vi "WPI_MotorControlSafetyCheck.vi"(0 "MotorControlDevRef":T1={"DeviceStatus"={"status"=FALSE, "code"=0, "source"=""}, "Type"=enum."PWM", "PWM"={"PWM Channel"=enum."Invalid", "DeadBand"={"Name"="", "maxPositivePwm"=0, "minPositivePwm"=0, "centerPwm"=0, "maxNegativePwm"=0, "minNegativePwm"=0, "angularRange"=0}}, "CAN"={"Device Number"=0, "SetOutput VI Ref"=variant(refnum<vi> refnum), "GetOutput VI Ref"=variant(refnum<vi> refnum), "Enable VI Ref"=variant(refnum<vi> refnum), "Disable VI Ref"=variant(refnum<vi> refnum), "Data"=variant}, "Invert"=FALSE, "DIO PWM"={"PWM \"Enable\" Channel"=enum."Invalid", "DIOChannel"=enum."Invalid", "PWM Rate"=0.0}}, 5 "menu":T6, 7 "VI Refnum":refnum<vi>, 9 "timeout (ms)":u32=100, 11 "error in (no error)":errorcluster) -> (15 "error out":errorcluster)   [LabVIEW 2025]
doc: "This subVI holds an array of DevRefs, timeout values, and latest update times. These values can be added, updated, tested, and removed.\n\nThis gets called by Open to add a set of values. It gets called by Drive to update the 'last update value'. It gets called by Close to remove a set of values.\n\nIt also gets called by Safety Test via the SafetyCheckEngine that runs as a background task called by the Start Communication loop to test all sets of values for a timeout condition.\n\nThis software is licensed. Open the labview\\readme\\WPI Robotics Library Open Source License.txt file for more information."
uses:
  <vilib>/Rock Robotics/WPI/SafetyOutput/WPI_SafetyOutputCheckMenu.ctl
  <vilib>/Rock Robotics/WPI/MotorControl/WPI_MotorControlDeviceRef.ctl
  <vilib>/Rock Robotics/WPI/MotorControl/WPI_MotorControlType.ctl
  <vilib>/Rock Robotics/SystemInterfaces/DIO/FPGA_DIOPWMChannel.ctl
  <vilib>/Rock Robotics/WPI/PWM/WPI_PWMDeadband.ctl
  <vilib>/Rock Robotics/SystemInterfaces/DIO/FPGA_DIOChannel.ctl
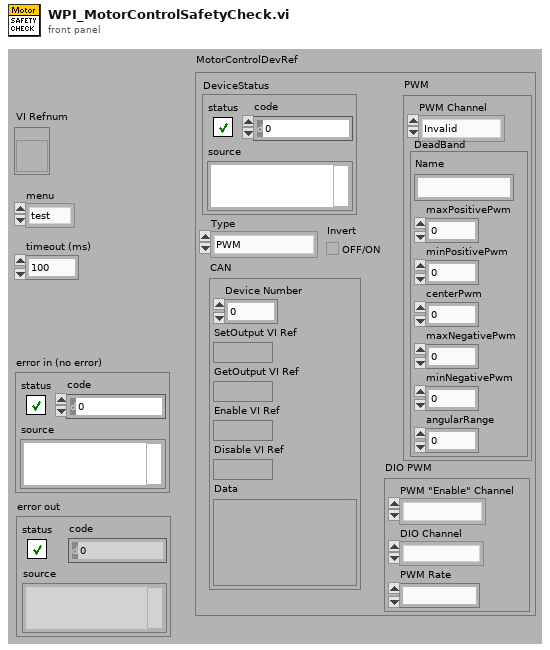
[diagram p1: front panel]
types:
  T1 = typedef "WPI_MotorControlDeviceRef.ctl" = cluster{"DeviceStatus":errorcluster, "Type":T2, "PWM":cluster{"PWM Channel":T3, "DeadBand":T4}, "CAN":cluster{"Device Number":u8, "SetOutput VI Ref":variant, "GetOutput VI Ref":variant, "Enable VI Ref":variant, "Disable VI Ref":variant, "Data":variant}, "Invert":bool, "DIO PWM":cluster{"PWM \"Enable\" Channel":T3, "DIOChannel":T5, "PWM Rate":dbl}}
  T2 = typedef "WPI_MotorControlType.ctl" = enum16{"PWM", "CAN", "DIO PWM"}
  T3 = typedef "FPGA_DIOPWMChannel.ctl" = enum8{"PWM 0", "PWM 1", "PWM 2", "PWM 3", "PWM 4", "PWM 5", "PWM 6", "PWM 7", "PWM 8", "PWM 9", "PWM MXP 0", "PWM MXP 1", "PWM MXP 2", "PWM MXP 3", "PWM MXP 4", "PWM MXP 5", "PWM MXP 6", "PWM MXP 7", "PWM MXP 8", "PWM MXP 9", "Invalid"}
  T4 = typedef "WPI_PWMDeadband.ctl" = cluster{"Name":string, "maxPositivePwm":i32, "minPositivePwm":i32, "centerPwm":i32, "maxNegativePwm":i32, "minNegativePwm":i32, "angularRange":u16}
  T5 = typedef "FPGA_DIOChannel.ctl" = enum8{"DIO 0", "DIO 1", "DIO 2", "DIO 3", "DIO 4", "DIO 5", "DIO 6", "DIO 7", "DIO 8", "DIO 9", "DIO MXP 0", "DIO MXP 1", "DIO MXP 2", "DIO MXP 3", "DIO MXP 4", "DIO MXP 5", "DIO MXP 6", "DIO MXP 7", "DIO MXP 8", "DIO MXP 9", "DIO MXP 10", "DIO MXP 11", "DIO MXP 12", "DIO MXP 13", "DIO MXP 14", "DIO MXP 15", "SPI Port CS1", "SPI Port CS2", "SPI Port CS3", "SPI Port MISO", "SPI Port MOSI", "Invalid"}
  T6 = typedef "WPI_SafetyOutputCheckMenu.ctl" = enum16{"test", "add", "remove", "update"}
  T7 = typedef "WPI_PWMDeviceRef.ctl" = cluster{"DeviceStatus":errorcluster, "PWM Channel":T3}
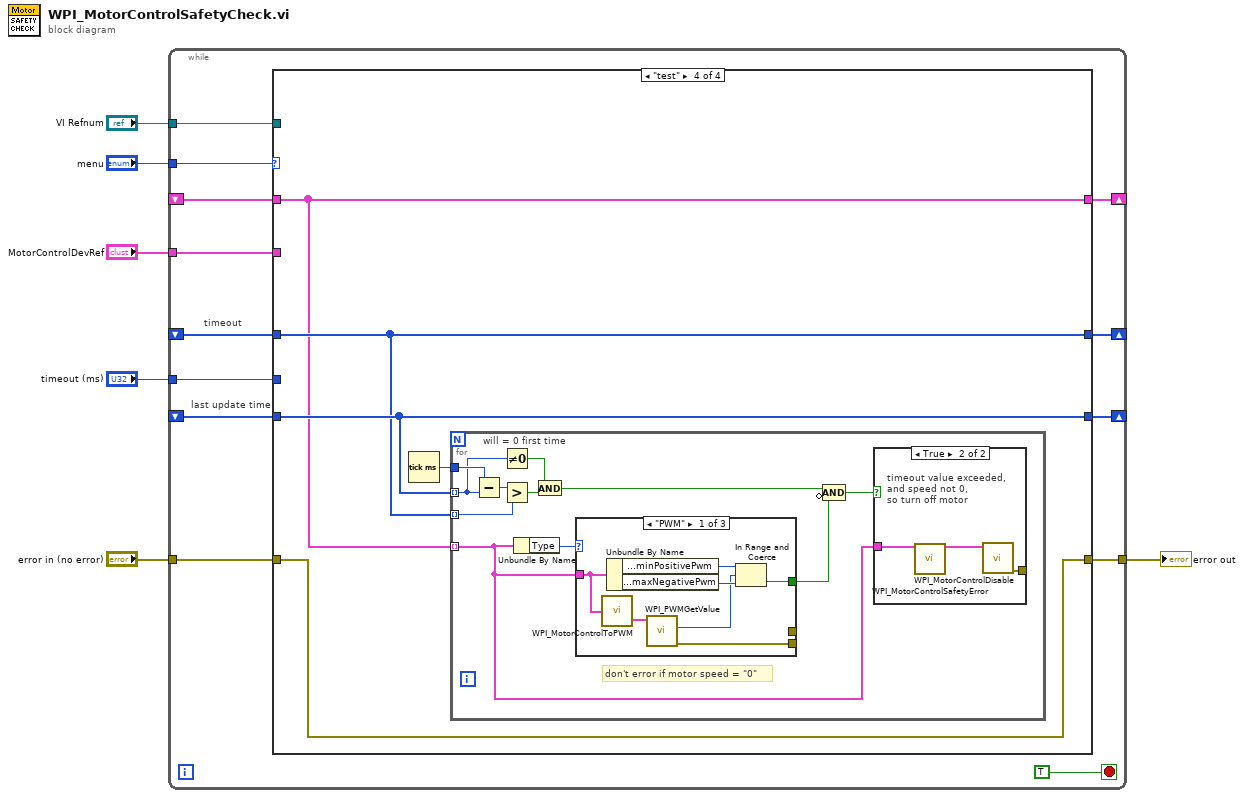
[diagram p0: block diagram]
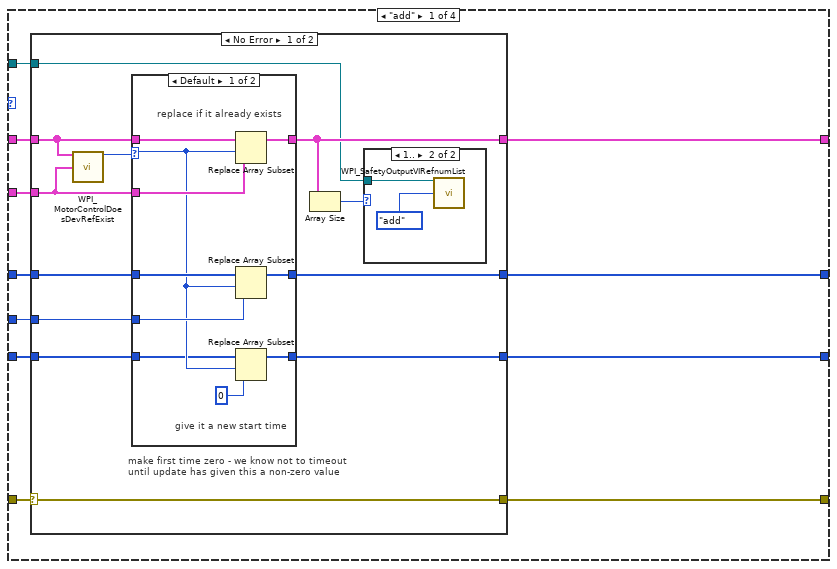
[diagram p2: hidden frame]
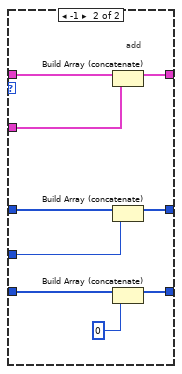
[diagram p4: hidden frame]
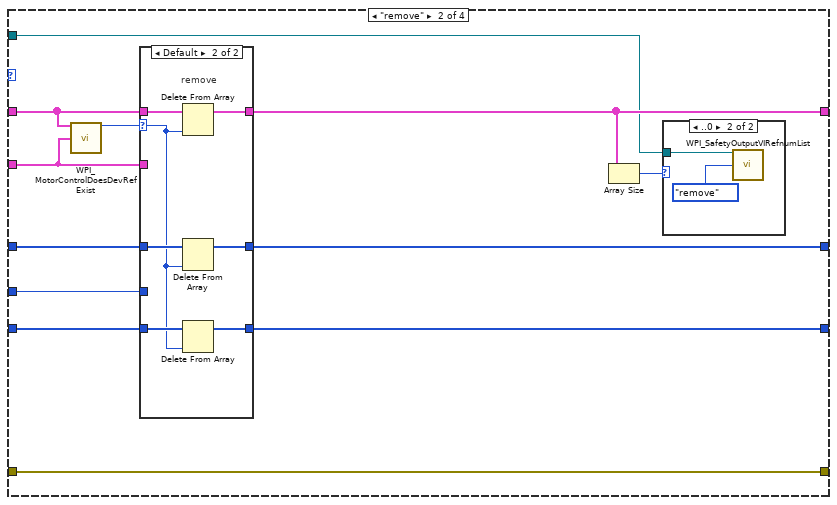
[diagram p6: hidden frame]
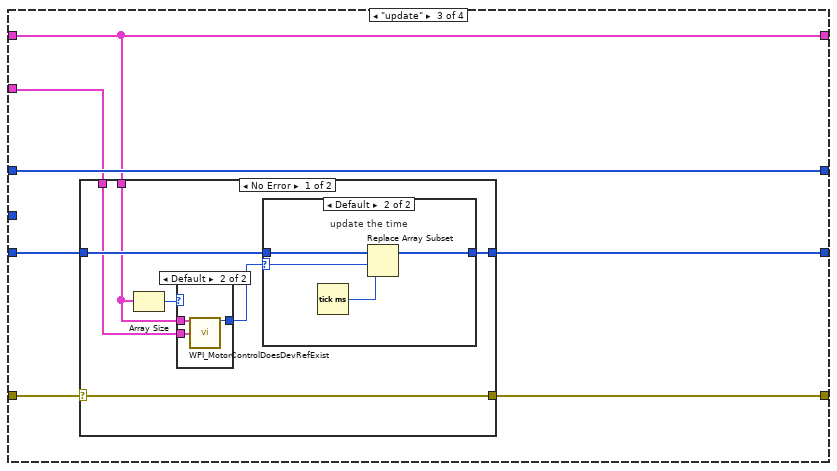
[diagram p9: hidden frame]
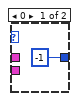
[diagram p10: hidden frame]
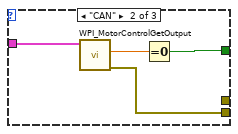
[diagram p13: hidden frame]
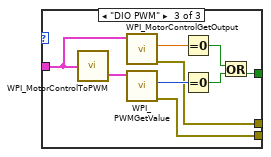
[diagram p14: hidden frame]
diagram:
  n1 = while {
    tunnel: "menu" -> [w18]
    shift-right: [w17] -> _
    shift-left: _ -> [w13]
    tunnel: "MotorControlDevRef" -> [w12]
    shift-right: [w14] -> _
    shift-left: _ -> [w16]
    tunnel: "timeout (ms)" -> [w15]
    shift-right: [w10] -> _
    shift-left: _ -> [w11]
    tunnel: "VI Refnum" -> [w9]
    tunnel: "error in (no error)" -> [w8]
    tunnel: [w7] -> w1
    stop <- TRUE stop-if-true
    # "last update time"
    # "timeout"
    n2 = case shown="\"test\"" w18 {
      tunnel: w13 -> [w30 w69 w93 w117]
      tunnel: [w23 w73 w93 w117] -> w17
      tunnel: w12 -> [w29 w68 w92 _]
      tunnel: w16 -> [w28 w79 w98 w119]
      tunnel: w15 -> [w27 w78 _ _]
      tunnel: [w26 w77 w98 w119] -> w14
      tunnel: w11 -> [w25 w76 w97 w120]
      tunnel: [w24 w75 w96 w120] -> w10
      tunnel: w9 -> [w22 w72 _ _]
      tunnel: w8 -> [w21 w71 w95 w118]
      tunnel: [w20 w71 w94 w118] -> w7
      frame "add" {
        n3 = case shown="No Error" w21 {
          selector: w21 -> [w34 w67]
          tunnel: w30 -> [w33 w66]
          tunnel: w29 -> [w31 _]
          tunnel: w28 -> [w42 w65]
          tunnel: w27 -> [w41 _]
          tunnel: [w40 w65] -> w26
          tunnel: w25 -> [w39 w64]
          tunnel: [w38 w64] -> w24
          tunnel: [w37 w66] -> w23
          tunnel: w22 -> [w36 _]
          tunnel: [w34 w67] -> w20
          frame No Error {
            # "make first time zero - we know not to timeout until update has given this a non-zero value"
            n4 = call <vilib>:"WPI_MotorControlDoesDevRefExist.vi"("MotorControlDeviceRefArray"=w33, "MotorControlDeviceRef"=w31) -> ("index"=w32:i32)  [unwired: 13 out]
            n5 = case shown="Default" w32 {
              selector: w32 -> [w47 _]
              tunnel: w33 -> [w54 w63]
              tunnel: [w53 w62] -> w37
              tunnel: w31 -> [w52 w61]
              tunnel: w42 -> [w51 w60]
              tunnel: w41 -> [w49 w59]
              tunnel: [w50 w58] -> w40
              tunnel: w39 -> [w46 w57]
              tunnel: [w45 w56] -> w38
              frame Default {
                # "give it a new start time"
                # "replace if it already exists"
                n6 = Replace Array Subset(array=w54, new element=w52, index=w47) -> (w53:T1[])
                n7 = Replace Array Subset(array=w51, new element=w49, index=w47) -> (w50:u32[])
                n8 = Replace Array Subset(array=w46, new element=u32 0 ("millisecond timer value"), index=w47) -> (w45:u32[])
              }
              frame -1 {
                # "add"
                n9 = Build Array (concatenate)(w63, w61) -> (w62:T1[])
                n10 = Build Array (concatenate)(w60, w59) -> (w58:u32[])
                n11 = Build Array (concatenate)(w57, u32 0 ("millisecond timer value")) -> (w56:u32[])
              }
            }
            n12 = Array Size(array=w37) -> (size(s)=w35:i32)
            n13 = case shown="1.." w35 {
              tunnel: w36 -> [_ w43]
              frame Default {
              }
              frame 1.. {
                n14 = call <vilib>:"WPI_SafetyOutputVIRefnumList.vi"("VI Refnum"=w43, "menu"=enum16{"read", "add", "remove"}."add") -> ()  [unwired: 14 out]
              }
            }
          }
          frame Error {
            # "do not add if there is an error"
          }
        }
      }
      frame "remove" {
        n15 = call <vilib>:"WPI_MotorControlDoesDevRefExist.vi"("MotorControlDeviceRefArray"=w69, "MotorControlDeviceRef"=w68) -> ("index"=w70:i32)  [unwired: 13 out]
        n16 = case shown="Default" w70 {
          selector: w70 -> [_ w85]
          tunnel: w69 -> [w84 w91]
          tunnel: [w84 w88] -> w73
          tunnel: w68 -> [_ _]
          tunnel: w79 -> [w83 w90]
          tunnel: w78 -> [_ _]
          tunnel: [w83 w87] -> w77
          tunnel: w76 -> [w82 w89]
          tunnel: [w82 w86] -> w75
          frame -1 {
            # "do nothing if it does not exist"
          }
          frame Default {
            # "remove"
            n17 = Delete From Array(array=w91, index=w85) -> (array with subset deleted=w88:T1[])  [unwired: 1 in, 1 out]
            n18 = Delete From Array(array=w90, index=w85) -> (array with subset deleted=w87:u32[])  [unwired: 1 in, 1 out]
            n19 = Delete From Array(array=w89, index=w85) -> (array with subset deleted=w86:u32[])  [unwired: 1 in, 1 out]
          }
        }
        n20 = Array Size(array=w73) -> (size(s)=w74:i32)
        n21 = case shown="..0" w74 {
          tunnel: w72 -> [_ w80]
          frame Default {
          }
          frame ..0 {
            n22 = call <vilib>:"WPI_SafetyOutputVIRefnumList.vi"("VI Refnum"=w80, "menu"=enum16{"read", "add", "remove"}."remove") -> ()  [unwired: 14 out]
          }
        }
      }
      frame "update" {
        n23 = case shown="No Error" w95 {
          selector: w95 -> [w103 w116]
          tunnel: w97 -> [w105 w115]
          tunnel: [w104 w115] -> w96
          tunnel: [w103 w116] -> w94
          tunnel: w93 -> [w100 _]
          tunnel: w92 -> [w99 _]
          frame No Error {
            n24 = Array Size(array=w100) -> (size(s)=w102:i32)
            n25 = case shown="Default" w102 {
              tunnel: w99 -> [_ w109]
              tunnel: [-1 w108] -> w101
              tunnel: w100 -> [_ w107]
              frame 0 {
              }
              frame Default {
                n26 = call <vilib>:"WPI_MotorControlDoesDevRefExist.vi"("MotorControlDeviceRefArray"=w107, "MotorControlDeviceRef"=w109) -> ("index"=w108:i32)  [unwired: 13 out]
              }
            }
            n27 = case shown="Default" w101 {
              selector: w101 -> [_ w111]
              tunnel: w105 -> [w110 w114]
              tunnel: [w110 w113] -> w104
              frame -1 {
                # "don't replace if it doesn't exist"
              }
              frame Default {
                # "update the time"
                n28 = Tick Count (ms)() -> (millisecond timer value=w112:u32)
                n29 = Replace Array Subset(array=w114, new element=w112, index=w111) -> (w113:u32[])
              }
            }
          }
          frame Error {
            # "do not update if there is an error"
          }
        }
      }
      frame "test" {
        n30 = Tick Count (ms)() -> (millisecond timer value=w121:u32)
        n31 = for {
          tunnel: w120 -> [w128] mode=indexing
          tunnel: w121 -> [w132]
          tunnel: w119 -> [w130] mode=indexing
          tunnel: w117 -> [w125] mode=indexing
          # "don't error if motor speed = \"0\""
          # "will = 0 first time"
          n32 = Subtract(x=w132, y=w128) -> (x-y=w131:u32)
          n33 = Not Equal To 0?(x=w128) -> (x != 0?=w127:bool)
          n34 = Greater?(x=w131, y=w130) -> (0:w129:bool)
          n35 = Unbundle By Name(w125) -> ("Type"=w126:T2)
          n36 = And(x=w127, y=w129) -> (x .and. y?=w123:bool)
          n37 = case shown="\"PWM\"" w126 {
            tunnel: w125 -> [w134 w141 w146]
            tunnel: [w135 w142 w148] -> w124
            tunnel: [w133 w140 w145] -> _
            tunnel: [_ _ w144] -> _
            frame "PWM" {
              n38 = call <vilib>:"WPI_MotorControlToPWM.vi"("MotorControlDeviceRef"=w134) -> ("PWMDeviceRef"=w139:T7)  [unwired: 1 out]
              n39 = Unbundle By Name(w134) -> ("PWM.DeadBand.minPositivePwm"=w137:i32, "PWM.DeadBand.maxNegativePwm"=w138:i32)
              n40 = call <vilib>:"WPI_PWMGetValue.vi"("PWMDeviceRef"=w139) -> ("error out"=w133:errorcluster, "Value"=w136:u16)  [unwired: 8 in, 1 out]
              n41 = In Range and Coerce(upper limit=w137, x=w136, lower limit=w138) -> (In Range?=w135:bool)  [unwired: 1 out]
            }
            frame "CAN" {
              n42 = call <vilib>:"WPI_MotorControlGetOutput.vi"("MotorControlDevRef"=w141) -> ("error out"=w140:errorcluster, "Output"=w143:dbl)  [unwired: 8 in, 1 out]
              n43 = Equal To 0?(x=w143) -> (x = 0?=w142:bool)
            }
            frame "DIO PWM" {
              n44 = call <vilib>:"WPI_MotorControlToPWM.vi"("MotorControlDeviceRef"=w146) -> ("PWMDeviceRef"=w152:T7)  [unwired: 1 out]
              n45 = call <vilib>:"WPI_MotorControlGetOutput.vi"("MotorControlDevRef"=w146) -> ("error out"=w144:errorcluster, "Output"=w149:dbl)  [unwired: 8 in, 1 out]
              n46 = call <vilib>:"WPI_PWMGetValue.vi"("PWMDeviceRef"=w152) -> ("error out"=w145:errorcluster, "Value"=w151:u16)  [unwired: 8 in, 1 out]
              n47 = Equal To 0?(x=w149) -> (x = 0?=w147:bool)
              n48 = Equal To 0?(x=w151) -> (x = 0?=w150:bool)
              n49 = Or(x=w147, y=w150) -> (x .or. y?=w148:bool)
            }
          }
          n50 = Compound Arithmetic op=AND(w123, invert w124) -> (w122:bool)
          n51 = case shown="True" w122 {
            tunnel: w125 -> [_ w155]
            tunnel: [_ w153] -> _
            frame False {
              # "do nothing"
            }
            frame True {
              # "timeout value exceeded, and speed not 0,\nso turn off motor"
              n52 = call <vilib>:"WPI_MotorControlSafetyError.vi"("MotorControlDevRef"=w155) -> ("MotorControlDevRef"=w154:T1)  [unwired: 14 out]
              n53 = call <vilib>:"WPI_MotorControlDisable.vi"("MotorControlDevRef"=w154) -> ("error out"=w153:errorcluster)  [unwired: 1 in, 9 out]
            }
          }
        }
      }
    }
  }
  "error out" <- w1
